vi "Send String.vi"(6 "error in (no error)":errorcluster, 8 "Bus In":refnum<class "Bus.lvclass">, 9 "Init in":refnum<class "Initialize.lvclass">) -> (0 "error out":errorcluster, 2 "Bus Out":refnum<class "Bus.lvclass">, 3 "Init out":refnum<class "Initialize.lvclass">)   [LabVIEW 2018, in "Initialize.lvclass"]
doc: "Initialize.lvclass:Send String.vi\n\nThis is the template for the Send String VI forthe Initialize class.\n\nInstrument Communication Module Version 1.0\nOctober, 2020 Original Code Consulting Davita Bird\n www.originalcode.com"
uses:
  Initialize.lvclass
  Bus/Bus.lvclass
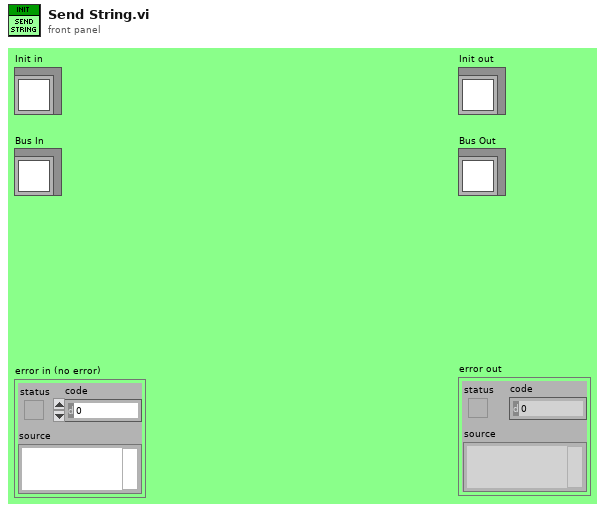
[diagram p1: front panel]
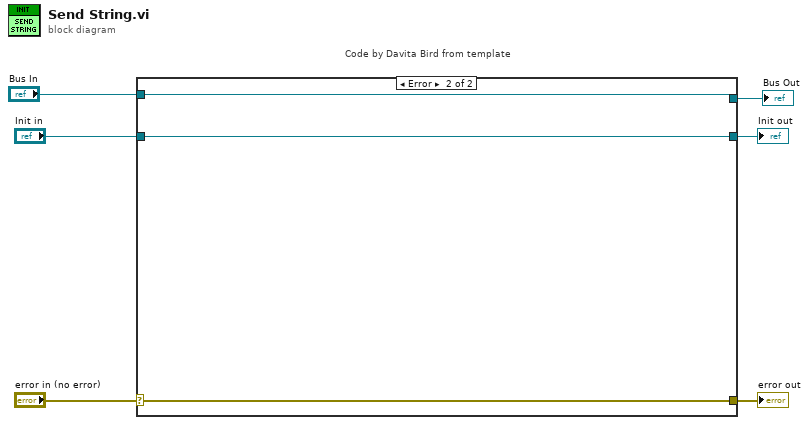
[diagram p0: block diagram]
diagram:
  n1 = case "Code by Davita Bird from template" shown="Error" "error in (no error)" {
    selector: "error in (no error)" -> [w8 w12]
    tunnel: [w8 w12] -> w5
    tunnel: [w9 w11] -> w3
    tunnel: "Init in" -> [w9 w11]
    tunnel: "Bus In" -> [w7 w10]
    tunnel: [w7 w10] -> w1
    frame No Error {
    }
    frame Error {
    }
  }
  "error out" <- w5
  "Init out" <- w3
  "Bus Out" <- w1
